vi "pco.camera_SaveImages_Example.vi"() -> ()   [LabVIEW 2020]
uses:
  <userlib>/PCO LabVIEW 5.0.0/pco.camera/Camera.lvclass
  <vilib>/picture/picture.llb/Draw 8-Bit Pixmap.vi
  <vilib>/picture/picture.llb/Draw True-Color Pixmap.vi
  <userlib>/PCO LabVIEW 5.0.0/pco.recorder/Recorder.lvlib
panel:
  out "colormap(U8)":u32[](array[numeric])
  out "Image(U16)":u16[][](graph)
  in  "Zoom [%]":i32(c297)=26
  out "Image":picture
  out "rawImage":u16[][](array[numeric])
  in  "data_format":T1(ring)=enum."Mono16"
  in  "Image Index":u32 max=999
  in  "saveImages":bool
  in  "SavePath":path
  out "Recorded Images":u32
  in  "Quit":bool
  in  "roiY1":u64=2 min=2 max=2160 step=1
  in  "roiX1":u64=2 min=2 max=2560 step=1
  in  "roiY0":u64=1 min=1 max=2159 step=1
  in  "roiX0":u64=1 min=1 max=2559 step=1
  out "Image Height":u16
  out "Image Width":u16
  in  "dwImgCount":u32=10 caption="Required Number of Images" max=4023
  out "Error":errorcluster {"code" format="%x"}
  # "This example shows how to record an image sequence and save all images to files (and an .avi) afterwards.\nIt is a good starting point for writing own applications with file saving\nBut it will not be fail save, i.e. doesnt react on errors, just handles them forward to the end\n\nUsage:\nSelect your required image count you want to record before you start the program.\nOnce started, the camera class will be initialized and images will be recorded automatically.\nWhen acquisition has finished you can read the images by index, crop them using the ROI parameters and select a file path.\nBy clicking save, the images are saved with the selected file format using the current active roi setting.\nThis also finishes the program and will force an exit of the camera class"
  # "pco.labview"
  # "Camera Setup"
  # "Recording Control"
  # "Parameters for image readout"
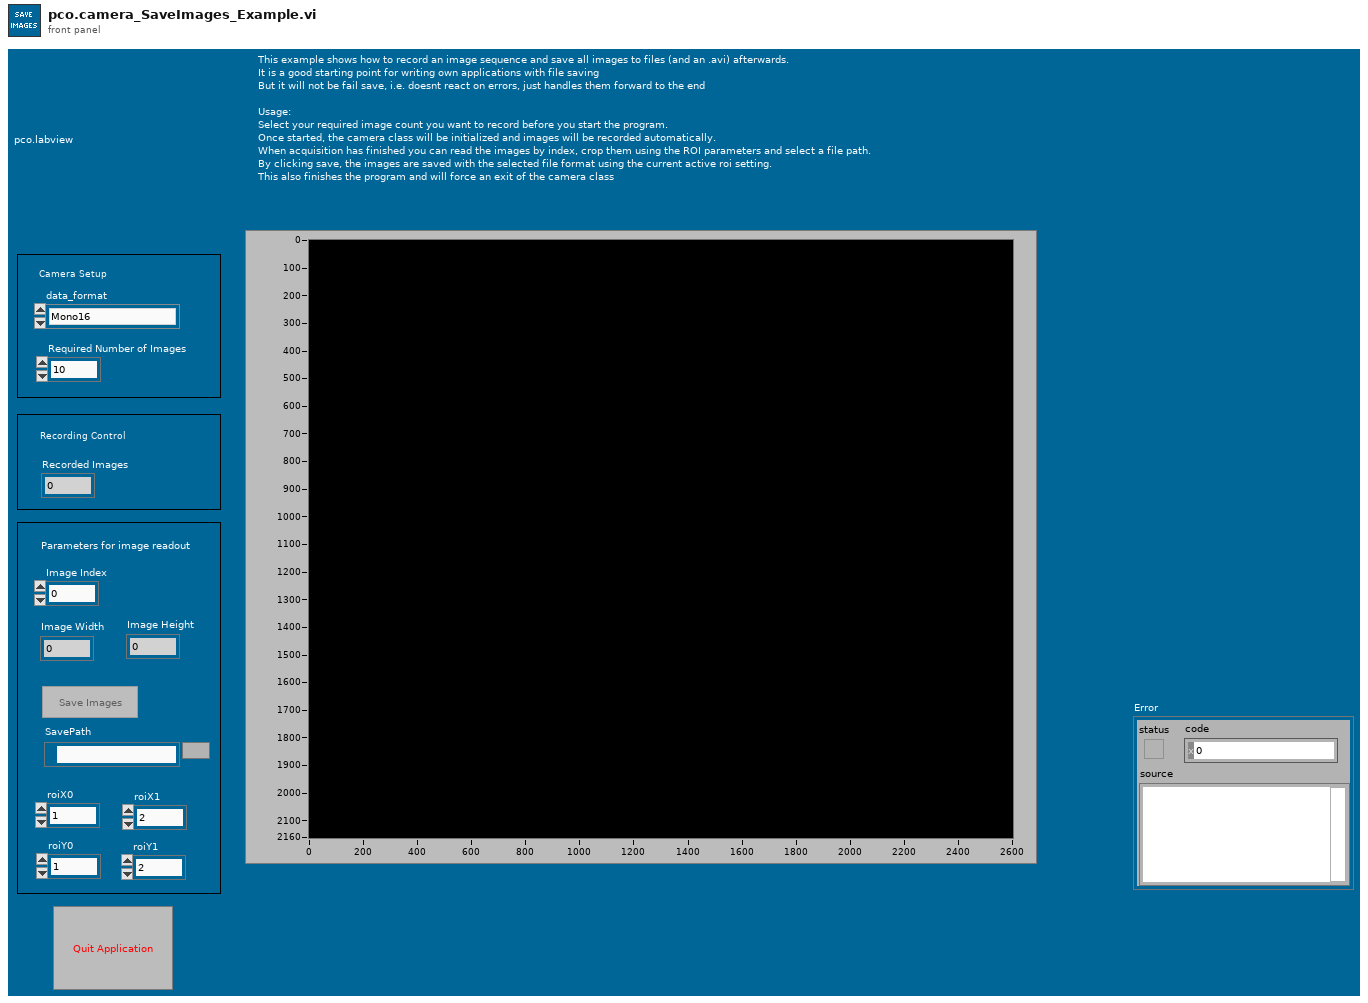
[diagram p1: front panel]
types:
  T1 = enum16{"Undefined", "Mono8", "Mono16", "BGRA8", "RGBA8", "BGRA16", "RGBA16", "CompressedMono8"}
  T2 = enum8{"Enabled", "Disabled", "Disabled and Grayed Out"}
  T3 = enum16{"sequence", "sequence non blocking", "ring buffer", "fifo", "sequence_dpcore", "sequence_non_blocking_dpcore", "ring_buffer_dpcore", "fifo_dpcore", "tif", "multitif", "pcoraw", "b16", "dicom", "multidicom"}
  T4 = typedef "Camera.lvclass/binning.ctl" = cluster{"vert":u16, "horz":u16}
  T5 = cluster{"exposure_time_s":dbl, "delay_time_s":dbl, "roi":cluster{"x0":u64, "y0":u64, "x1":u64, "y1":u64}, "timestamp_mode":u16, "pixelrate":u32, "trigger_mode":u16, "acquire_mode":u16, "metadata_mode":u16, "noisefilter_mode":u16, "binning":T4}
  T6 = cluster{"wVersion":u16, "dwIMAGE_COUNTER":u32, "dwIMAGE_TIME_US":u32, "lvTimestamp":timestamp, "bIMAGE_TIME_STATUS":u8, "wEXPOSURE_TIME_BASE":u16, "dwEXPOSURE_TIME":u32, "dwFRAMERATE_MILLIHZ":u32, "sSENSOR_TEMPERATURE":i16, "wIMAGE_SIZE_X":u16, "wIMAGE_SIZE_Y":u16, "bBINNING_X":u8, "bBINNING_Y":u8, "dwSENSOR_READOUT_FREQUENCY":u32, "wSENSOR_CONV_FACTOR":u16, "dwCAMERA_SERIAL_NO":u32, "wCAMERA_TYPE":u16, "bBIT_RESOLUTION":u8, "bSYNC_STATUS":u8, "wDARK_OFFSET":u16, "bTRIGGER_MODE":u8, "bDOUBLE_IMAGE_MODE":u8, "bCAMERA_SYNC_MODE":u8, "bIMAGE_TYPE":u8, "wCOLOR_PATTERN":u16, "wCAMERA_SUBTYPE":u16, "dwEVENT_NUMBER":u32, "wIMAGE_SIZE_X_Offset":u16, "wIMAGE_SIZE_Y_Offset":u16}[]
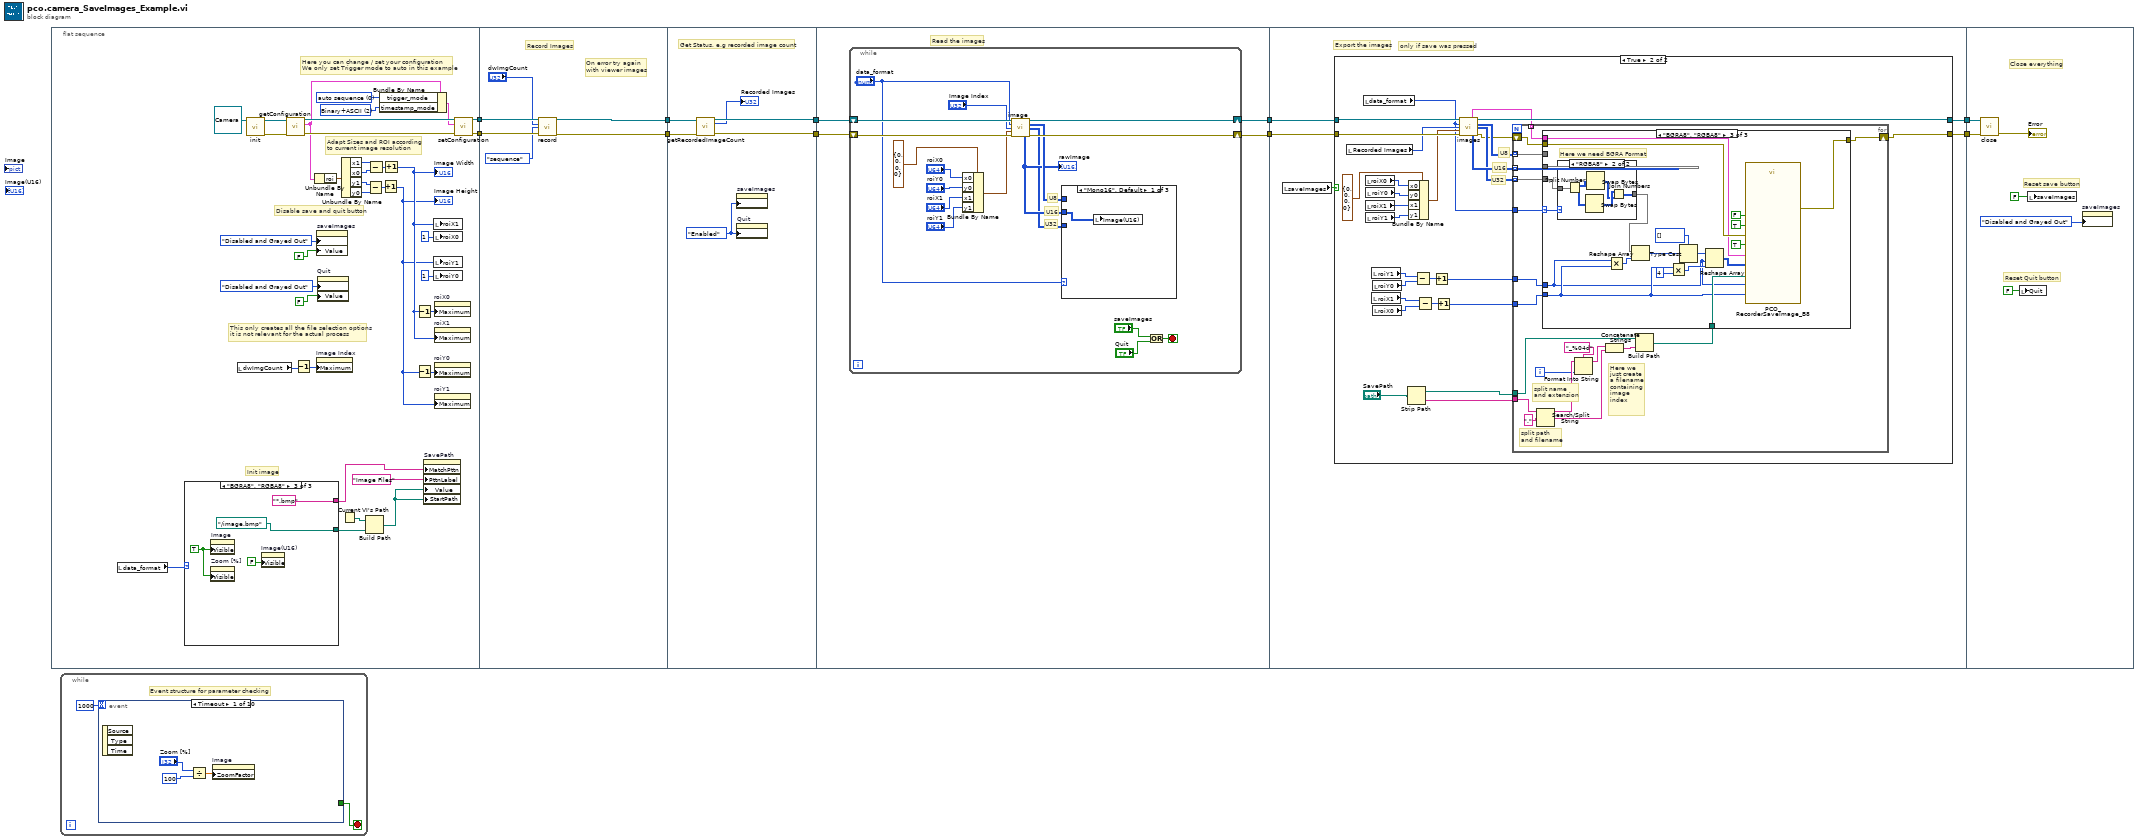
[diagram p0: block diagram]
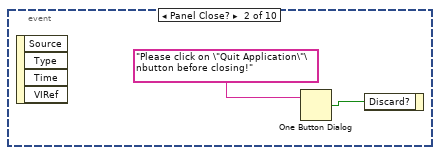
[diagram p2: hidden frame]
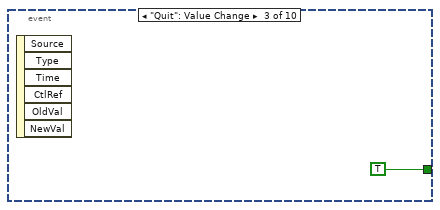
[diagram p3: hidden frame]
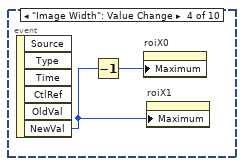
[diagram p4: hidden frame]
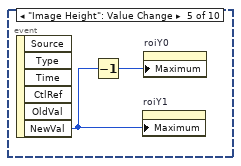
[diagram p5: hidden frame]
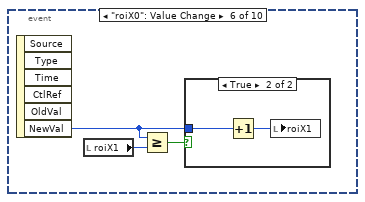
[diagram p6: hidden frame]
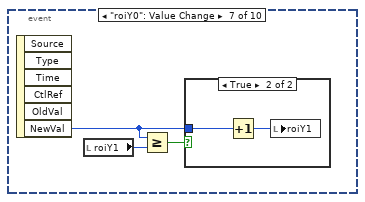
[diagram p8: hidden frame]
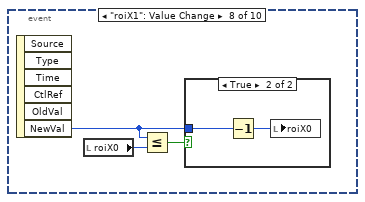
[diagram p10: hidden frame]
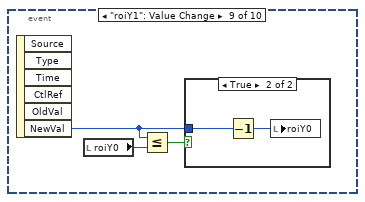
[diagram p12: hidden frame]
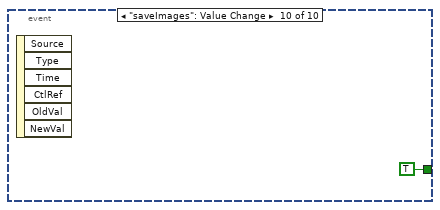
[diagram p14: hidden frame]
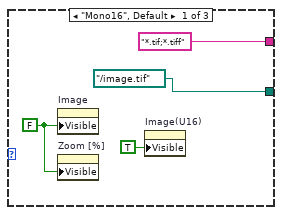
[diagram p15: hidden frame]
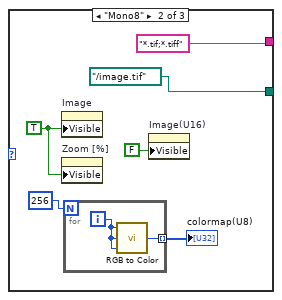
[diagram p16: hidden frame]
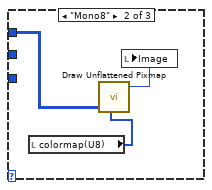
[diagram p17: hidden frame]
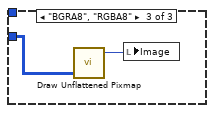
[diagram p18: hidden frame]
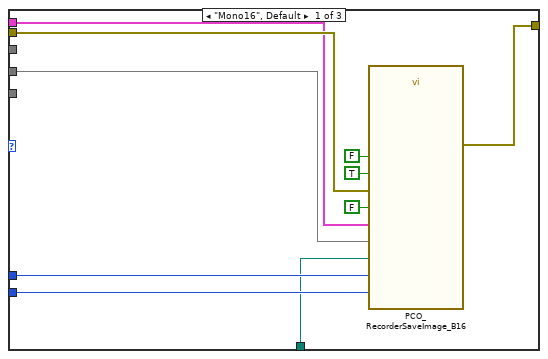
[diagram p20: hidden frame]
diagram:
  n1 = flat-sequence {
    tunnel: [w37] -> w10
    tunnel: [w36] -> w9
    tunnel: w10 -> [w68]
    tunnel: w9 -> [w67]
    tunnel: [w65] -> w8
    tunnel: [w64] -> w7
    tunnel: w8 -> [w74]
    tunnel: w7 -> [w73]
    tunnel: [w72] -> w6
    tunnel: [w71] -> w5
    tunnel: w6 -> [w77]
    tunnel: w5 -> [w78]
    tunnel: [w76] -> w4
    tunnel: [w75] -> w2
    tunnel: w4 -> [w106]
    tunnel: [w105] -> w3
    tunnel: w2 -> [w104]
    tunnel: [w103] -> w1
    tunnel: w3 -> [w208]
    tunnel: w1 -> [w207]
    frame #0 {
      w21 = u16 2 items=["OFF", "Binary", "Binary+ASCII", "ASCII"] ("TimestampMode")
      w43 = u16 0 items=["auto sequence"=0, "software trigger"=1, "external exposure start & software trigger"=2, "external exposure control"=3, "external synchronized"=4, "fast external exposure control"=5, "external CDS control"=6, "slow external exposure control"=7, "external synchronized HDSDI"=258] ("TriggerMode")
      # "Init image"
      # "This only creates all the file selection options\nit is not relevant for the actual process"
      # "Adapt Sizes and ROI according\nto current image resolution"
      # "Disable save and quit button"
      # "Here you can change / set your configuration\nWe only set Trigger mode to auto in this example"
      n2 = local read "data_format"() -> (w13:T1)
      n3 = case shown="\"BGRA8\", \"RGBA8\"" w13 {
        tunnel: [path "../image.tif" ("SavePath") path "../image.tif" ("SavePath") path "../image.bmp" ("SavePath")] -> w12
        tunnel: ["*.tif;*.tiff" ("pattern (all files)") "*.tif;*.tiff" ("pattern (all files)") "*.bmp" ("pattern (all files)")] -> w11
        frame "Mono16", Default {
          w49 = FALSE ("Visible")
          n4 = property on="Image" class="Pict"("Visible"=w49) -> ()  [unwired: 2 in, 2 out]
          n5 = property on="Zoom [%]" class="Scroll (strict)"("Visible"=w49) -> ()  [unwired: 2 in, 2 out]
          n6 = property on="Image(U16)" class="IntGraph (strict)"("Visible"=TRUE) -> ()  [unwired: 2 in, 2 out]
        }
        frame "Mono8" {
          w55 = TRUE ("Visible")
          n7 = property on="Image" class="Pict"("Visible"=w55) -> ()  [unwired: 2 in, 2 out]
          n8 = property on="Zoom [%]" class="Scroll (strict)"("Visible"=w55) -> ()  [unwired: 2 in, 2 out]
          n9 = for {
            N: 256 -> [_]
            tunnel: [w57] -> w54 mode=indexing
            i -> [w58]
            n10 = call <vilib>:"RGB to Color.vi"("B"=w58, "G"=w58, "R"=w58) -> ("Color"=w57:u32)
          }
          "colormap(U8)" <- w54
          n11 = property on="Image(U16)" class="IntGraph (strict)"("Visible"=FALSE) -> ()  [unwired: 2 in, 2 out]
        }
        frame "BGRA8", "RGBA8" {
          w61 = TRUE ("Visible")
          n12 = property on="Image" class="Pict"("Visible"=w61) -> ()  [unwired: 2 in, 2 out]
          n13 = property on="Zoom [%]" class="Scroll (strict)"("Visible"=w61) -> ()  [unwired: 2 in, 2 out]
          n14 = property on="Image(U16)" class="IntGraph (strict)"("Visible"=FALSE) -> ()  [unwired: 2 in, 2 out]
        }
      }
      n15 = local read "dwImgCount"() -> (w14:u32)
      n16 = call-dynamic "init.vi"("Camera in"=refnum<class "Camera.lvclass"> refnum ("PCOCamera in")) -> ("Camera out"=w45:refnum<class "Camera.lvclass">, "error out"=w44:errorcluster)  [unwired: 8 in]
      n17 = call-dynamic "getConfiguration.vi"("error in (no error)"=w44, "Camera in"=w45) -> ("error out"=w41:errorcluster, "configuration"=w31:T5, "Camera out"=w42:refnum<class "Camera.lvclass">)  [unwired: 7 in]
      n18 = Decrement(x=w14) -> (x-1=w15:u32)
      n19 = Unbundle By Name(w31) -> ("roi"=w30:cluster{"x0":u64, "y0":u64, "x1":u64, "y1":u64})
      n20 = property on="Image Index" class="DigNum (strict)"("Maximum"=w15) -> ()  [unwired: 2 in, 2 out]
      n21 = property on="saveImages" class="Bool (strict)"("DisabledEnum"=T2."Disabled and Grayed Out" ("Disabled"), "Value"=FALSE ("Stop")) -> ()  [unwired: 2 in, 2 out]
      n22 = property on="Quit" class="Bool (strict)"("DisabledEnum"=T2."Disabled and Grayed Out" ("Disabled"), "Value"=FALSE ("Stop")) -> ()  [unwired: 2 in, 2 out]
      n23 = Current VI's Path() -> (path=w18:path)
      n24 = Unbundle By Name(w30) -> ("x1"=w28:u64, "x0"=w29:u64, "y1"=w26:u64, "y0"=w27:u64)
      n25 = Build Path(base path=w18, name or relative path=w12) -> (appended path=w16:path)
      n26 = Subtract(x=w26, y=w27) -> (x-y=w24:u64)
      n27 = Subtract(x=w28, y=w29) -> (x-y=w25:u64)
      n28 = Bundle By Name(cluster=w31, "trigger_mode"=w43, "timestamp_mode"=w21) -> (w40:T5)
      n29 = Increment(x=w24) -> (x+1=w22:u64)
      "Image Height" <- w22
      n30 = Increment(x=w25) -> (x+1=w23:u64)
      "Image Width" <- w23
      n31 = Decrement(x=w23) -> (x-1=w33:u64)
      n32 = Decrement(x=w22) -> (x-1=w32:u64)
      n33 = property on="SavePath" class="Path"("MatchPttn"=w11, "PttnLabel"="Image Files" ("pattern label"), "Value"=w16, "StartPath"=w16) -> ()  [unwired: 2 in, 2 out]
      n34 = local write "roiX1"(w23) -> ()
      n35 = local write "roiX0"(u16 1 ("roiY0")) -> ()
      n36 = local write "roiY1"(w22) -> ()
      n37 = local write "roiY0"(u16 1 ("roiY0")) -> ()
      n38 = property on="roiX0" class="DigNum (strict)"("Maximum"=w33) -> ()  [unwired: 2 in, 2 out]
      n39 = property on="roiX1" class="DigNum (strict)"("Maximum"=w23) -> ()  [unwired: 2 in, 2 out]
      n40 = property on="roiY0" class="DigNum (strict)"("Maximum"=w32) -> ()  [unwired: 2 in, 2 out]
      n41 = property on="roiY1" class="DigNum (strict)"("Maximum"=w22) -> ()  [unwired: 2 in, 2 out]
      n42 = call-dynamic "setConfiguration.vi"("error in (no error)"=w41, "configuration"=w40, "Camera in"=w42) -> ("error out"=w36:errorcluster, "Camera out"=w37:refnum<class "Camera.lvclass">)  [unwired: 7 in]
    }
    frame #1 {
      # "On error try again \nwith viewer images"
      # "Record Images"
      n43 = call-dynamic "record.vi"("Camera in"=w68, "num_images"="dwImgCount", "record_mode"=T3."sequence", "error in (no error)"=w67) -> ("Camera out"=w65:refnum<class "Camera.lvclass">, "error out"=w64:errorcluster)  [unwired: 10 in]
    }
    frame #2 {
      w69 = T2."Enabled" ("Disabled")
      # "Get Status, e.g recorded image count"
      n44 = call-dynamic "getRecordedImageCount.vi"("Camera in"=w74, "error in (no error)"=w73) -> ("Camera out"=w72:refnum<class "Camera.lvclass">, "recorded_image_count"=→"Recorded Images":u32, "error out"=w71:errorcluster)  [unwired: 11 in]
      n45 = property on="saveImages" class="Bool (strict)"("DisabledEnum"=w69) -> ()  [unwired: 2 in, 2 out]
      n46 = property on="Quit" class="Bool (strict)"("DisabledEnum"=w69) -> ()  [unwired: 2 in, 2 out]
    }
    frame #3 {
      # "Read the images"
      n47 = while {
        shift-right: [w94] -> w76
        shift-left: w77 -> [w96]
        shift-right: [w89] -> w75
        shift-left: w78 -> [w95]
        stop <- w87 stop-if-true
        # "U32"
        # "U16"
        # "U8"
        n48 = Bundle By Name(cluster=cluster{"x0":u64, "y0":u64, "x1":u64, "y1":u64} {"x0"=0, "y0"=0, "x1"=0, "y1"=0} ("roi"), "x0"="roiX0", "y0"="roiY0", "x1"="roiX1", "y1"="roiY1") -> (w85:cluster{"x0":u64, "y0":u64, "x1":u64, "y1":u64})
        n49 = call-dynamic "image.vi"("Camera in"=w96, "data_format"="data_format", "image_index"="Image Index", "roi"=w85, "error in (no error)"=w95) -> ("Camera out"=w94:refnum<class "Camera.lvclass">, "image (U8)"=w82:u8[][], "image (U32)"=w80:u32[][], "raw_image (U16)"=w81:u16[][], "error out"=w89:errorcluster)  [unwired: 3 in, 3 out]
        "rawImage" <- w81
        n50 = case shown="\"Mono16\", Default" "data_format" {
          tunnel: w80 -> [_ _ w102]
          tunnel: w82 -> [_ w100 _]
          tunnel: w81 -> [w97 _ _]
          frame "Mono16", Default {
            n51 = local write "Image(U16)"(w97) -> ()
          }
          frame "Mono8" {
            n52 = local read "colormap(U8)"() -> (w99:u32[])
            n53 = call-poly <vilib>:"Draw Unflattened Pixmap.vi"("data"=w100, "color table"=w99) -> ("new picture"=w98:picture)  [unwired: 7 in]
            n54 = local write "Image"(w98) -> ()
          }
          frame "BGRA8", "RGBA8" {
            n55 = call-poly <vilib>:"Draw Unflattened Pixmap.vi"("data (RGB format)"=w102) -> ("new picture"=w101:picture)  [unwired: 8 in]
            n56 = local write "Image"(w101) -> ()
          }
        }
        n57 = Or(x="saveImages", y="Quit") -> (x .or. y?=w87:bool)
      }
    }
    frame #4 {
      # "only if save was pressed"
      # "Export the images"
      n58 = local read "saveImages"() -> (w107:bool)
      n59 = case shown="True" w107 {
        tunnel: w106 -> [w109 w136]
        tunnel: [w109 w125] -> w105
        tunnel: w104 -> [w108 w137]
        tunnel: [w108 w119] -> w103
        frame False {
        }
        frame True {
          # "U32"
          # "U16"
          # "U8"
          n60 = local read "Recorded Images"() -> (w129:u32)
          n61 = local read "data_format"() -> (w124:T1)
          n62 = local read "roiX0"() -> (w134:u64)
          n63 = local read "roiX1"() -> (w132:u64)
          n64 = local read "roiY0"() -> (w133:u64)
          n65 = local read "roiY1"() -> (w131:u64)
          n66 = local read "roiY1"() -> (w116:u64)
          n67 = local read "roiX1"() -> (w114:u64)
          n68 = local read "roiY0"() -> (w115:u64)
          n69 = local read "roiX0"() -> (w113:u64)
          n70 = Strip Path(path="SavePath") -> (stripped path=w121:path, name=w122:string)
          n71 = Bundle By Name(cluster=cluster{"x0":u64, "y0":u64, "x1":u64, "y1":u64} {"x0"=0, "y0"=0, "x1"=0, "y1"=0} ("roi"), "x0"=w134, "y0"=w133, "x1"=w132, "y1"=w131) -> (w130:cluster{"x0":u64, "y0":u64, "x1":u64, "y1":u64})
          n72 = Subtract(x=w116, y=w115) -> (x-y=w118:u64)
          n73 = Subtract(x=w114, y=w113) -> (x-y=w117:u64)
          n74 = Increment(x=w118) -> (x+1=w111:u64)
          n75 = Increment(x=w117) -> (x+1=w112:u64)
          n76 = call-dynamic "images.vi"("Camera in"=w136, "data_format"=w124, "image_count"=w129, "roi"=w130, "error in (no error)"=w137) -> ("meta_data_list"=w110:T6, "Camera out"=w125:refnum<class "Camera.lvclass">, "image_list (U8)"=w128:u8[][][], "image_list (U32)"=w126:u32[][][], "raw_image_list (U16)"=w127:u16[][][], "error out"=w120:errorcluster)  [unwired: 3 in, 2 out]
          n77 = for {
            tunnel: w128 -> [w156] mode=indexing
            tunnel: w127 -> [w155] mode=indexing
            tunnel: w126 -> [w139] mode=indexing
            tunnel: w124 -> [w147]
            tunnel: w122 -> [w146]
            tunnel: w121 -> [w145]
            shift-right: [w143] -> w119
            shift-left: w120 -> [w144]
            tunnel: w112 -> [w140]
            tunnel: w111 -> [w141]
            tunnel: w110 -> [w142] mode=indexing
            i -> [w148]
            # "Here we \njust create\na filename\ncontaining\nimage \nindex"
            # "split path \nand filename"
            # "split name \nand extension"
            n78 = Search/Split String(string=w146, search string/char (-)=".") -> (substring before match=w152:string, match + rest of string=w153:string)  [unwired: 1 in, 1 out]
            n79 = Format Into String(format string="_%04d", initial string=w152, w148) -> (resulting string=w154:string)  [unwired: 1 in, 1 out]
            n80 = Concatenate Strings(w154, w153) -> (w149:string)
            n81 = Build Path(base path=w145, name or relative path=w149) -> (appended path=w138:path)
            n82 = case shown="\"BGRA8\", \"RGBA8\"" w147 {
              selector: w147 -> [_ _ w178]
              tunnel: w156 -> [_ w173 _]
              tunnel: w155 -> [w161 _ _]
              tunnel: w141 -> [w163 w171 w177]
              tunnel: w140 -> [w162 w170 w179]
              tunnel: w144 -> [w160 w172 w192]
              tunnel: [w159 w169 w191] -> w143
              tunnel: w142 -> [w158 w168 w190]
              tunnel: w139 -> [_ _ w188]
              tunnel: w138 -> [w157 w167 w189]
              frame "Mono16", Default {
                n83 = call <userlib>:"PCO_RecorderSaveImage_B16.vi"("pImgBuf"=w161, "wWidth"=w162, "wHeight"=w163, "szFilePath"=w157, "error in (no error)"=w160, "isColor"=FALSE, "bIsBitmap"=FALSE, "PCO_METADATA_STRUCT"=w158, "bOverwrite"=TRUE) -> ("error out"=w159:errorcluster)  [unwired: 9 in, 1 out]
              }
              frame "Mono8" {
                n84 = call <userlib>:"PCO_RecorderSaveImage_B8.vi"("pImgBuf"=w173, "wWidth"=w170, "wHeight"=w171, "szFilePath"=w167, "error in (no error)"=w172, "isColor"=FALSE, "bIsBitmap"=FALSE, "PCO_METADATA_STRUCT"=w168, "bOverwrite"=TRUE) -> ("error out"=w169:errorcluster)  [unwired: 9 in, 1 out]
              }
              frame "BGRA8", "RGBA8" {
                # "Here we need BGRA Format"
                n85 = case shown="\"RGBA8\"" w178 {
                  tunnel: w188 -> [w196 w202]
                  tunnel: [w196 w197] -> w180
                  frame Default {
                  }
                  frame "RGBA8" {
                    n86 = Split Number(x=w202) -> (hi(x)=w201:u16[][], lo(x)=w200:u16[][])
                    n87 = Swap Bytes(anything=w200) -> (byte swapped=w199:u16[][])
                    n88 = Swap Bytes(anything=w201) -> (byte swapped=w198:u16[][])
                    n89 = Join Numbers(hi=w199, lo=w198) -> ((hi.lo)=w197:u32[][])
                  }
                }
                n90 = Multiply(x=w177, y=w179) -> (x*y=w182:u64)
                n91 = Reshape Array(w180, w182) -> (w181:u32[])
                n92 = Multiply(x=w179, y=u64 4) -> (x*y=w186:u64)
                n93 = Type Cast(type=u8[] [] ("image_list (U32)"), x=w181) -> (*(type *) &x=w187:u8[])
                n94 = Reshape Array(w187, w177, w186) -> (w183:u8[][])
                n95 = call <userlib>:"PCO_RecorderSaveImage_B8.vi"("pImgBuf"=w183, "wWidth"=w179, "wHeight"=w177, "szFilePath"=w189, "error in (no error)"=w192, "isColor"=TRUE, "bIsBitmap"=FALSE, "PCO_METADATA_STRUCT"=w190, "bOverwrite"=TRUE) -> ("error out"=w191:errorcluster)  [unwired: 9 in, 1 out]
              }
            }
          }
        }
      }
    }
    frame #5 {
      # "Reset Quit button"
      # "Close everything"
      # "Reset save button"
      n96 = call-dynamic "close.vi"("error in (no error)"=w207, "Camera in"=w208) -> ("error out"=→"Error":errorcluster)  [unwired: 9 in]
      n97 = local write "Quit"(FALSE ("Stop")) -> ()
      n98 = local write "saveImages"(FALSE ("Stop")) -> ()
      n99 = property on="saveImages" class="Bool (strict)"("DisabledEnum"=T2."Disabled and Grayed Out" ("Disabled")) -> ()  [unwired: 2 in, 2 out]
    }
  }
  n100 = while {
    stop <- w209 stop-if-true
    # "Event structure for parameter checking"
    n101 = event shown="[0] Timeout" {
      selector: _ -> [_ _ _ _ _ _ _ _ _ _]
      dyn-events: _ -> [_ _ _ _ _ _ _ _ _ _]
      timeout: 1000 -> [_ _ _ _ _ _ _ _ _ _]
      tunnel: [_ _ TRUE _ _ _ _ _ _ TRUE] -> w209
      event Timeout {
        n102 = event-data() -> ()  [unwired: 1 in, 3 out]
        n103 = Divide(x="Zoom [%]", y=100 ("Zoom [%]")) -> (x/y=w213:dbl)
        n104 = property on="Image" class="Pict"("ZoomFactor"=w213) -> ()  [unwired: 2 in, 2 out]
      }
      event Panel Close? {
        n105 = event-data() -> ()  [unwired: 1 in, 4 out]
        n106 = One Button Dialog(message="Please click on \"Quit Application\"\nbutton before closing!") -> (true=w214:bool)  [unwired: 1 in]
        n107 = event-data("Discard?"=w214) -> ()  [unwired: 1 in, 1 out]
      }
      event "Quit": Value Change {
        n108 = event-data() -> ()  [unwired: 1 in, 6 out]
      }
      event "Image Width": Value Change {
        n109 = event-data() -> ("NewVal"=w217:u16)  [unwired: 1 in, 5 out]
        n110 = Decrement(x=w217) -> (x-1=w218:u16)
        n111 = property on="roiX0" class="DigNum (strict)"("Maximum"=w218) -> ()  [unwired: 2 in, 2 out]
        n112 = property on="roiX1" class="DigNum (strict)"("Maximum"=w217) -> ()  [unwired: 2 in, 2 out]
      }
      event "Image Height": Value Change {
        n113 = event-data() -> ("NewVal"=w219:u16)  [unwired: 1 in, 5 out]
        n114 = Decrement(x=w219) -> (x-1=w220:u16)
        n115 = property on="roiY1" class="DigNum (strict)"("Maximum"=w219) -> ()  [unwired: 2 in, 2 out]
        n116 = property on="roiY0" class="DigNum (strict)"("Maximum"=w220) -> ()  [unwired: 2 in, 2 out]
      }
      event "roiX0": Value Change {
        n117 = event-data() -> ("NewVal"=w221:u64)  [unwired: 1 in, 5 out]
        n118 = local read "roiX1"() -> (w223:u64)
        n119 = Greater Or Equal?(x=w221, y=w223) -> (x >= y?=w222:bool)
        n120 = case shown="True" w222 {
          tunnel: w221 -> [_ w225]
          frame False {
          }
          frame True {
            n121 = Increment(x=w225) -> (x+1=w224:u64)
            n122 = local write "roiX1"(w224) -> ()
          }
        }
      }
      event "roiY0": Value Change {
        n123 = event-data() -> ("NewVal"=w226:u64)  [unwired: 1 in, 5 out]
        n124 = local read "roiY1"() -> (w228:u64)
        n125 = Greater Or Equal?(x=w226, y=w228) -> (x >= y?=w227:bool)
        n126 = case shown="True" w227 {
          tunnel: w226 -> [_ w230]
          frame False {
          }
          frame True {
            n127 = Increment(x=w230) -> (x+1=w229:u64)
            n128 = local write "roiY1"(w229) -> ()
          }
        }
      }
      event "roiX1": Value Change {
        n129 = event-data() -> ("NewVal"=w231:u64)  [unwired: 1 in, 5 out]
        n130 = local read "roiX0"() -> (w233:u64)
        n131 = Less Or Equal?(x=w231, y=w233) -> (x <= y?=w232:bool)
        n132 = case shown="True" w232 {
          tunnel: w231 -> [_ w235]
          frame False {
          }
          frame True {
            n133 = Decrement(x=w235) -> (x-1=w234:u64)
            n134 = local write "roiX0"(w234) -> ()
          }
        }
      }
      event "roiY1": Value Change {
        n135 = event-data() -> ("NewVal"=w236:u64)  [unwired: 1 in, 5 out]
        n136 = local read "roiY0"() -> (w238:u64)
        n137 = Less Or Equal?(x=w236, y=w238) -> (x <= y?=w237:bool)
        n138 = case shown="True" w237 {
          tunnel: w236 -> [_ w240]
          frame False {
          }
          frame True {
            n139 = Decrement(x=w240) -> (x-1=w239:u64)
            n140 = local write "roiY0"(w239) -> ()
          }
        }
      }
      event "saveImages": Value Change {
        n141 = event-data() -> ()  [unwired: 1 in, 6 out]
      }
    }
  }
